vi "PCO_RecorderSaveImage_B16.vi"(0 "pImgBuf":u16[][](array[numeric])=array1x4097[4097 elements], 1 "wWidth":u16, 2 "wHeight":u16, 3 "szFilePath":path, 5 "error in (no error)":errorcluster {"code" format="%x"}, 6 "isColor":bool, 8 "bIsBitmap":bool, 9 "PCO_METADATA_STRUCT":T1={"wVersion"=65535, "dwIMAGE_COUNTER"=0, "dwIMAGE_TIME_US"=0, "lvTimestamp"=timestamp(0 s since 1904-01-01), "bIMAGE_TIME_STATUS"=0, "wEXPOSURE_TIME_BASE"=0, "dwEXPOSURE_TIME"=0, "dwFRAMERATE_MILLIHZ"=0, "sSENSOR_TEMPERATURE"=0, "wIMAGE_SIZE_X"=0, "wIMAGE_SIZE_Y"=0, "bBINNING_X"=0, "bBINNING_Y"=0, "dwSENSOR_READOUT_FREQUENCY"=0, "wSENSOR_CONV_FACTOR"=0, "dwCAMERA_SERIAL_NO"=0, "wCAMERA_TYPE"=0, "bBIT_RESOLUTION"=0, "bSYNC_STATUS"=0, "wDARK_OFFSET"=0, "bTRIGGER_MODE"=0, "bDOUBLE_IMAGE_MODE"=0, "bCAMERA_SYNC_MODE"=0, "bIMAGE_TYPE"=0, "wCOLOR_PATTERN"=0, "wCAMERA_SUBTYPE"=0, "dwEVENT_NUMBER"=0, "wIMAGE_SIZE_X_Offset"=0, "wIMAGE_SIZE_Y_Offset"=0}, 10 "bOverwrite":bool) -> (14 "ErrorMessage":i32 format="%x", 19 "error out":errorcluster {"code" format="%x"})   [LabVIEW 2019, in "Recorder.lvlib"]
doc: "int WINAPI PCO_RecorderSaveImage(void* pImgBuf, WORD wWidth, WORD wHeight, const char* cFileType, bool bIsBitmap, const char* szFilePath, bool bOverwrite, PCO_METADATA_STRUCT* strMetadata);"
uses:
  Recorder.lvlib
  pco.sdk/Structures/Structures.lvlib
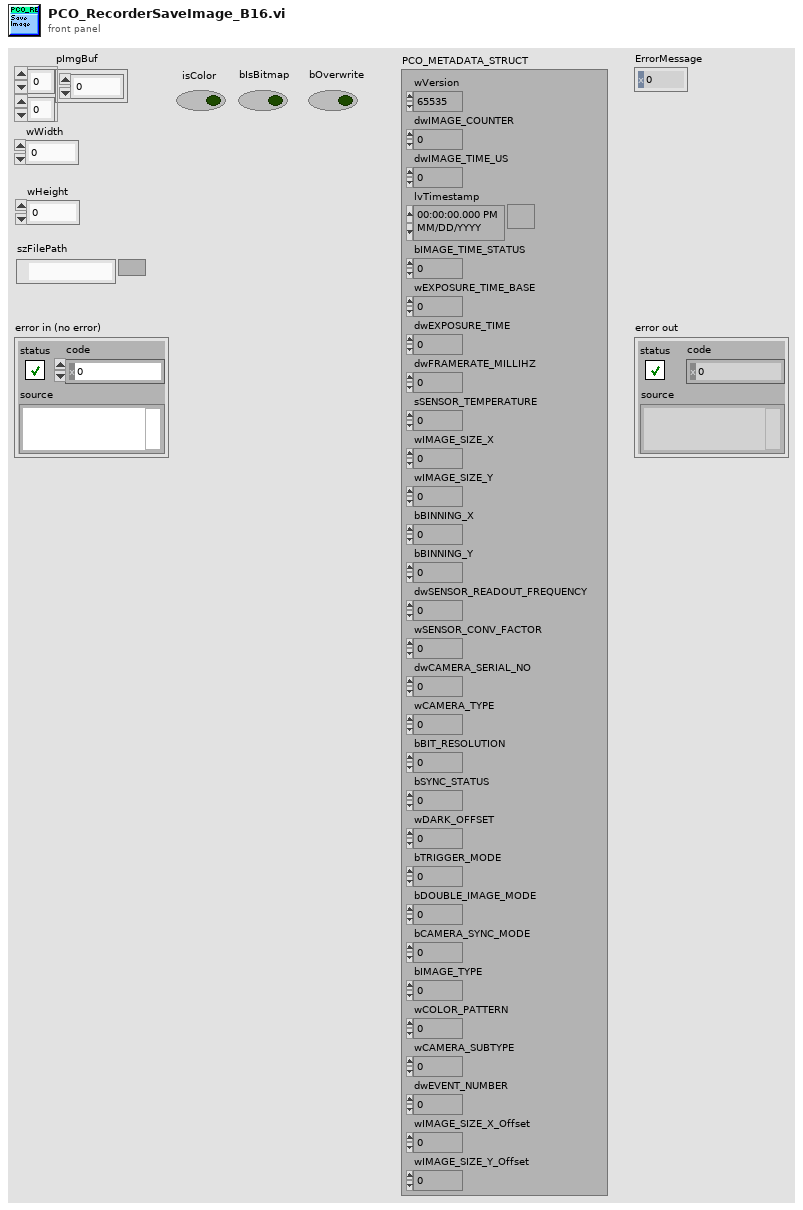
[diagram p1: front panel]
types:
  T1 = cluster{"wVersion":u16, "dwIMAGE_COUNTER":u32, "dwIMAGE_TIME_US":u32, "lvTimestamp":timestamp, "bIMAGE_TIME_STATUS":u8, "wEXPOSURE_TIME_BASE":u16, "dwEXPOSURE_TIME":u32, "dwFRAMERATE_MILLIHZ":u32, "sSENSOR_TEMPERATURE":i16, "wIMAGE_SIZE_X":u16, "wIMAGE_SIZE_Y":u16, "bBINNING_X":u8, "bBINNING_Y":u8, "dwSENSOR_READOUT_FREQUENCY":u32, "wSENSOR_CONV_FACTOR":u16, "dwCAMERA_SERIAL_NO":u32, "wCAMERA_TYPE":u16, "bBIT_RESOLUTION":u8, "bSYNC_STATUS":u8, "wDARK_OFFSET":u16, "bTRIGGER_MODE":u8, "bDOUBLE_IMAGE_MODE":u8, "bCAMERA_SYNC_MODE":u8, "bIMAGE_TYPE":u8, "wCOLOR_PATTERN":u16, "wCAMERA_SUBTYPE":u16, "dwEVENT_NUMBER":u32, "wIMAGE_SIZE_X_Offset":u16, "wIMAGE_SIZE_Y_Offset":u16}
  T2 = typedef "LVDateTimeRec.ctl" = cluster{"fractional second":dbl, "second":i32, "minute":i32, "hour":i32, "day of month":i32, "month":i32, "year":i32, "day of week":i32, "day of year":i32, "DST":i32}
  T3 = cluster{"wSize":u16, "wVersion":u16, "bIMAGE_COUNTER_BCD":cluster{u8, u8, u8, u8}, "bIMAGE_TIME_US_BCD":cluster{u8, u8, u8}, "bIMAGE_TIME_SEC_BCD":u8, "bIMAGE_TIME_MIN_BCD":u8, "bIMAGE_TIME_HOUR_BCD":u8, "bIMAGE_TIME_DAY_BCD":u8, "bIMAGE_TIME_MON_BCD":u8, "bIMAGE_TIME_YEAR_BCD":u8, "bIMAGE_TIME_STATUS":u8, "wEXPOSURE_TIME_BASE":u16, "dwEXPOSURE_TIME":u32, "dwFRAMERATE_MILLIHZ":u32, "sSENSOR_TEMPERATURE":i16, "wIMAGE_SIZE_X":u16, "wIMAGE_SIZE_Y":u16, "bBINNING_X":u8, "bBINNING_Y":u8, "dwSENSOR_READOUT_FREQUENCY":u32, "wSENSOR_CONV_FACTOR":u16, "dwCAMERA_SERIAL_NO":u32, "wCAMERA_TYPE":u16, "bBIT_RESOLUTION":u8, "bSYNC_STATUS":u8, "wDARK_OFFSET":u16, "bTRIGGER_MODE":u8, "bDOUBLE_IMAGE_MODE":u8, "bCAMERA_SYNC_MODE":u8, "bIMAGE_TYPE":u8, "wCOLOR_PATTERN":u16, "wCAMERA_SUBTYPE":u16, "dwEVENT_NUMBER":u32, "wIMAGE_SIZE_X_Offset":u16, "wIMAGE_SIZE_Y_Offset":u16}
  T4 = enum16{"big-endian, network order", "native, host order", "little-endian"}
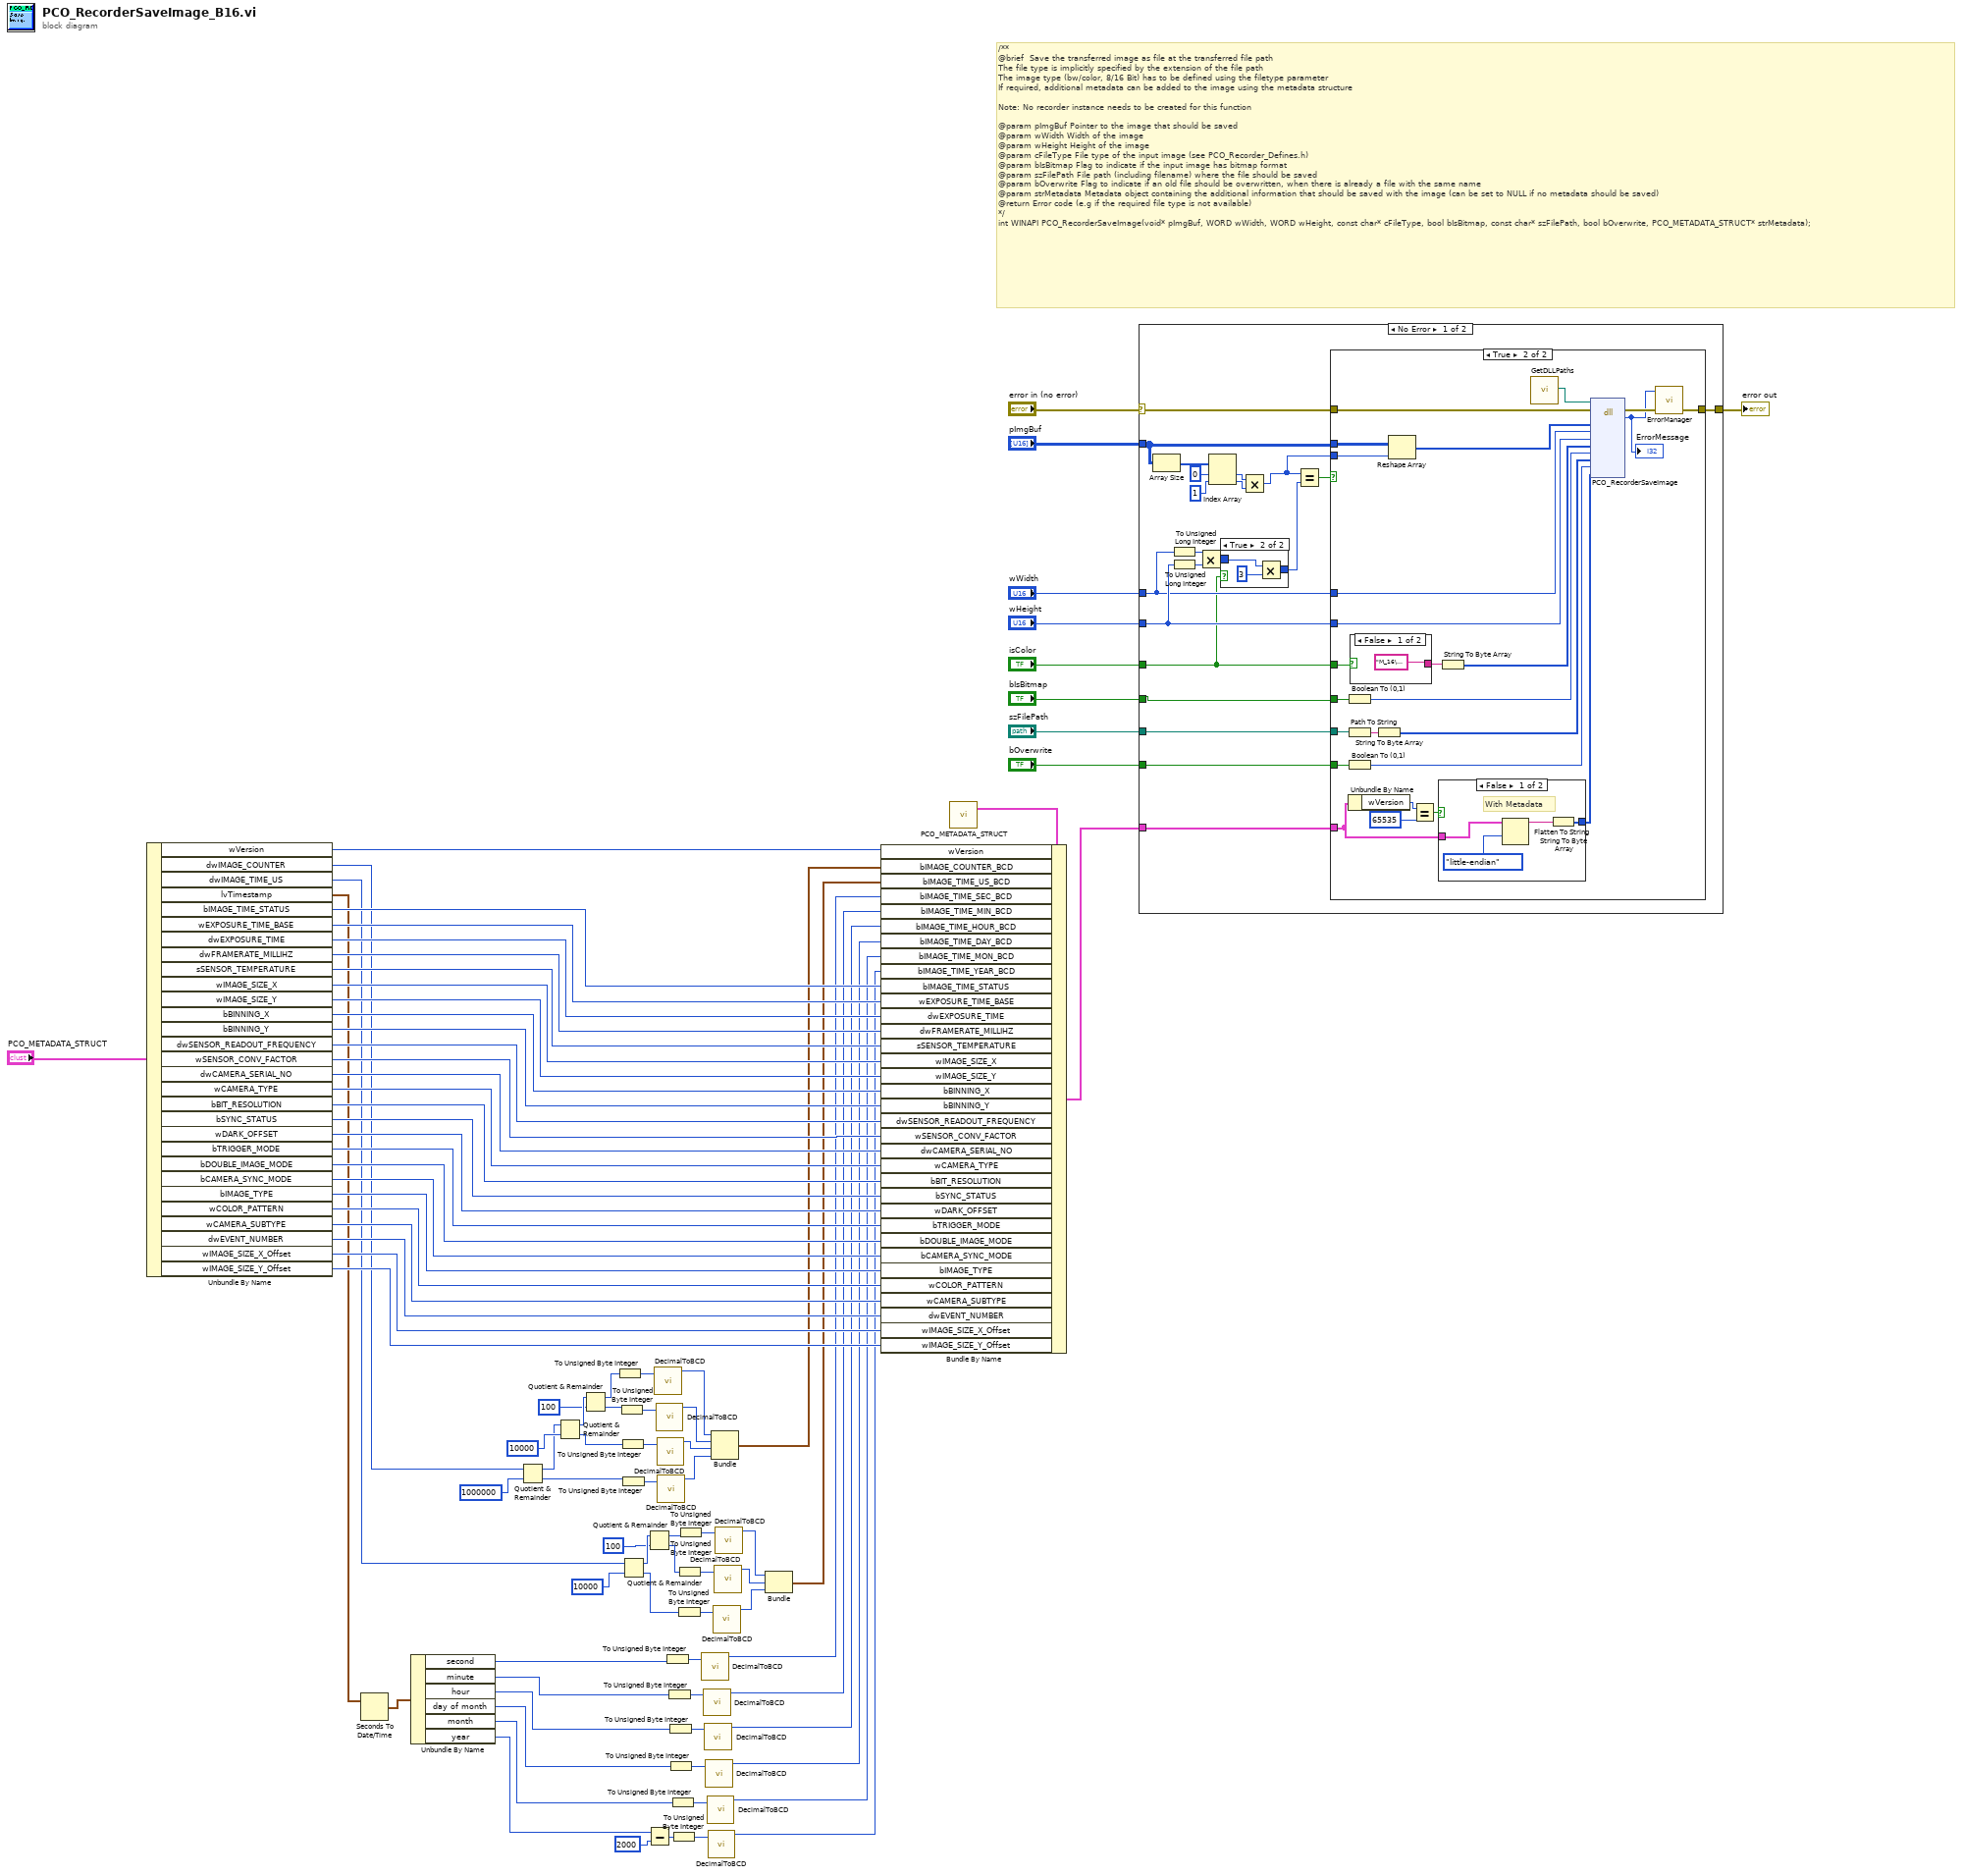
[diagram p0: block diagram]
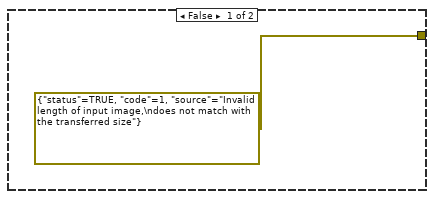
[diagram p3: hidden frame]
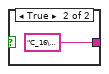
[diagram p4: hidden frame]
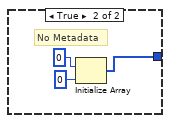
[diagram p5: hidden frame]
diagram:
  # "/**\n@brief  Save the transferred image as file at the transferred file path\nThe file type is implicitly specified by the extension of the file path\nThe image type (bw/color, 8/16 Bit) has to be defined using the filetype parameter\nIf required, additional metadata can be added to the image using the metadata structure\n\nNote: No recorder instance needs to be created for this function\n\n@param pImgBuf Pointer to the image that should be saved\n@param wWidth Width of the image\n@param wHeight Height of the image\n@param cFileType File type of the input image (see PCO_Recorder_Defines.h)\n@param bIsBitmap Flag to indicate if the input image has bitmap format\n@param szFilePath File path (including filename) where the file should be saved\n@param bOverwrite Flag to indicate if an old file should be overwritten, when there is already a file with the same name\n@param strMetadata Metadata object containing the additional information that should be saved with the image (can be set to NULL if no metadata should be saved)\n@return Error code (e.g if the required file type is not available)\n*/\nint WINAPI PCO_RecorderSaveImage(void* pImgBuf, WORD wWidth, WORD wHeight, const char* cFileType, bool bIsBitmap, const char* szFilePath, bool bOverwrite, PCO_METADATA_STRUCT* strMetadata);"
  n1 = Unbundle By Name("PCO_METADATA_STRUCT") -> ("wVersion"=w83:u16, "dwIMAGE_COUNTER"=w17:u32, "dwIMAGE_TIME_US"=w22:u32, "lvTimestamp"=w57:timestamp, "bIMAGE_TIME_STATUS"=w71:u8, "wEXPOSURE_TIME_BASE"=w58:u16, "dwEXPOSURE_TIME"=w59:u32, "dwFRAMERATE_MILLIHZ"=w60:u32, "sSENSOR_TEMPERATURE"=w61:i16, "wIMAGE_SIZE_X"=w62:u16, "wIMAGE_SIZE_Y"=w63:u16, "bBINNING_X"=w64:u8, "bBINNING_Y"=w65:u8, "dwSENSOR_READOUT_FREQUENCY"=w66:u32, "wSENSOR_CONV_FACTOR"=w67:u16, "dwCAMERA_SERIAL_NO"=w68:u32, "wCAMERA_TYPE"=w69:u16, "bBIT_RESOLUTION"=w70:u8, "bSYNC_STATUS"=w72:u8, "wDARK_OFFSET"=w73:u16, "bTRIGGER_MODE"=w74:u8, "bDOUBLE_IMAGE_MODE"=w75:u8, "bCAMERA_SYNC_MODE"=w76:u8, "bIMAGE_TYPE"=w77:u8, "wCOLOR_PATTERN"=w78:u16, "wCAMERA_SUBTYPE"=w79:u16, "dwEVENT_NUMBER"=w80:u32, "wIMAGE_SIZE_X_Offset"=w81:u16, "wIMAGE_SIZE_Y_Offset"=w82:u16)
  n2 = Seconds To Date/Time(time stamp (now)=w57) -> (date time rec=w56:T2)  [unwired: 1 in]
  n3 = Unbundle By Name(w56) -> ("second"=w55:i32, "minute"=w52:i32, "hour"=w47:i32, "day of month"=w46:i32, "month"=w45:i32, "year"=w42:i32)
  n4 = Quotient & Remainder(x=w17, y=u32 1000000 ("x")) -> (x-y*floor(x/y)=w16:u32, floor(x/y)=w11:u32)
  n5 = Quotient & Remainder(x=w16, y=u32 10000 ("x")) -> (x-y*floor(x/y)=w20:u32, floor(x/y)=w10:u32)
  n6 = Quotient & Remainder(x=w20, y=u32 100 ("x")) -> (x-y*floor(x/y)=w8:u32, floor(x/y)=w9:u32)
  n7 = To Unsigned Byte Integer(number=w8) -> (unsigned 8bit integer=w15:u8)
  n8 = To Unsigned Byte Integer(number=w9) -> (unsigned 8bit integer=w14:u8)
  n9 = To Unsigned Byte Integer(number=w10) -> (unsigned 8bit integer=w13:u8)
  n10 = To Unsigned Byte Integer(number=w11) -> (unsigned 8bit integer=w12:u8)
  n11 = Quotient & Remainder(x=w22, y=u32 10000 ("x")) -> (x-y*floor(x/y)=w34:u32, floor(x/y)=w27:u32)
  n12 = Quotient & Remainder(x=w34, y=u32 100 ("x")) -> (x-y*floor(x/y)=w31:u32, floor(x/y)=w29:u32)
  n13 = Subtract(x=w42, y=2000) -> (x-y=w43:i32)
  n14 = call "DecimalToBCD.vi"("U8"=w15) -> ("BCD"=w7:u8)  [unwired: 10 in]
  n15 = call "DecimalToBCD.vi"("U8"=w14) -> ("BCD"=w6:u8)  [unwired: 10 in]
  n16 = call "DecimalToBCD.vi"("U8"=w13) -> ("BCD"=w5:u8)  [unwired: 10 in]
  n17 = call "DecimalToBCD.vi"("U8"=w12) -> ("BCD"=w4:u8)  [unwired: 10 in]
  n18 = To Unsigned Byte Integer(number=w55) -> (unsigned 8bit integer=w54:u8)
  n19 = To Unsigned Byte Integer(number=w52) -> (unsigned 8bit integer=w53:u8)
  n20 = To Unsigned Byte Integer(number=w47) -> (unsigned 8bit integer=w51:u8)
  n21 = To Unsigned Byte Integer(number=w46) -> (unsigned 8bit integer=w48:u8)
  n22 = To Unsigned Byte Integer(number=w45) -> (unsigned 8bit integer=w49:u8)
  n23 = To Unsigned Byte Integer(number=w43) -> (unsigned 8bit integer=w50:u8)
  n24 = To Unsigned Byte Integer(number=w27) -> (unsigned 8bit integer=w28:u8)
  n25 = To Unsigned Byte Integer(number=w29) -> (unsigned 8bit integer=w30:u8)
  n26 = To Unsigned Byte Integer(number=w31) -> (unsigned 8bit integer=w32:u8)
  n27 = call "DecimalToBCD.vi"("U8"=w54) -> ("BCD"=w36:u8)  [unwired: 10 in]
  n28 = call "DecimalToBCD.vi"("U8"=w53) -> ("BCD"=w37:u8)  [unwired: 10 in]
  n29 = call "DecimalToBCD.vi"("U8"=w51) -> ("BCD"=w38:u8)  [unwired: 10 in]
  n30 = call "DecimalToBCD.vi"("U8"=w48) -> ("BCD"=w39:u8)  [unwired: 10 in]
  n31 = call "DecimalToBCD.vi"("U8"=w49) -> ("BCD"=w40:u8)  [unwired: 10 in]
  n32 = call "DecimalToBCD.vi"("U8"=w50) -> ("BCD"=w41:u8)  [unwired: 10 in]
  n33 = Bundle("BCD"=w7, "BCD"=w6, "BCD"=w5, "BCD"=w4) -> (w3:cluster{"BCD":u8, "BCD":u8, "BCD":u8, "BCD":u8})  [unwired: 1 in]
  n34 = call "DecimalToBCD.vi"("U8"=w28) -> ("BCD"=w24:u8)  [unwired: 10 in]
  n35 = call "DecimalToBCD.vi"("U8"=w30) -> ("BCD"=w25:u8)  [unwired: 10 in]
  n36 = call "DecimalToBCD.vi"("U8"=w32) -> ("BCD"=w26:u8)  [unwired: 10 in]
  n37 = Bundle("BCD"=w26, "BCD"=w25, "BCD"=w24) -> (w23:cluster{"BCD":u8, "BCD":u8, "BCD":u8})  [unwired: 1 in]
  n38 = call "PCO_METADATA_STRUCT.vi"() -> ("PCO_METADATA_STRUCT_Raw"=w84:T3)  [unwired: 4 in, 3 out]
  n39 = Bundle By Name(cluster=w84, "wVersion"=w83, "bIMAGE_COUNTER_BCD"=w3, "bIMAGE_TIME_US_BCD"=w23, "bIMAGE_TIME_SEC_BCD"=w36, "bIMAGE_TIME_MIN_BCD"=w37, "bIMAGE_TIME_HOUR_BCD"=w38, "bIMAGE_TIME_DAY_BCD"=w39, "bIMAGE_TIME_MON_BCD"=w40, "bIMAGE_TIME_YEAR_BCD"=w41, "bIMAGE_TIME_STATUS"=w71, "wEXPOSURE_TIME_BASE"=w58, "dwEXPOSURE_TIME"=w59, "dwFRAMERATE_MILLIHZ"=w60, "sSENSOR_TEMPERATURE"=w61, "wIMAGE_SIZE_X"=w62, "wIMAGE_SIZE_Y"=w63, "bBINNING_X"=w64, "bBINNING_Y"=w65, "dwSENSOR_READOUT_FREQUENCY"=w66, "wSENSOR_CONV_FACTOR"=w67, "dwCAMERA_SERIAL_NO"=w68, "wCAMERA_TYPE"=w69, "bBIT_RESOLUTION"=w70, "bSYNC_STATUS"=w72, "wDARK_OFFSET"=w73, "bTRIGGER_MODE"=w74, "bDOUBLE_IMAGE_MODE"=w75, "bCAMERA_SYNC_MODE"=w76, "bIMAGE_TYPE"=w77, "wCOLOR_PATTERN"=w78, "wCAMERA_SUBTYPE"=w79, "dwEVENT_NUMBER"=w80, "wIMAGE_SIZE_X_Offset"=w81, "wIMAGE_SIZE_Y_Offset"=w82) -> (w1:T3)
  n40 = case shown="No Error" "error in (no error)" {
    selector: "error in (no error)" -> [w113 w154]
    tunnel: "pImgBuf" -> [w112 _]
    tunnel: "wWidth" -> [w95 _]
    tunnel: "wHeight" -> [w96 _]
    tunnel: "bIsBitmap" -> [w106 _]
    tunnel: [w114 w154] -> w89
    tunnel: "szFilePath" -> [w107 _]
    tunnel: "bOverwrite" -> [w108 _]
    tunnel: "isColor" -> [w94 _]
    tunnel: w1 -> [w109 _]
    frame No Error {
      n41 = Array Size(array=w112) -> (size(s)=w105:i32[])
      n42 = To Unsigned Long Integer(number=w95) -> (unsigned 32bit integer=w98:u32)
      n43 = To Unsigned Long Integer(number=w96) -> (unsigned 32bit integer=w97:u32)
      n44 = Multiply(x=w98, y=w97) -> (x*y=w111:u32)
      n45 = Index Array(array=w105, index #1=0 ("index"), index #2=1 ("index")) -> (element #1=w103:i32, element #2=w101:i32)
      n46 = case shown="True" w94 {
        tunnel: w111 -> [w115 w118]
        tunnel: [w115 w116] -> w100
        frame False {
        }
        frame True {
          n47 = Multiply(x=w118, y=u16 3) -> (x*y=w116:u32)
        }
      }
      n48 = Multiply(x=w103, y=w101) -> (x*y=w99:i32)
      n49 = Equal?(x=w99, y=w100) -> (x = y?=w110:bool)
      n50 = case shown="True" w110 {
        tunnel: w112 -> [_ w122]
        tunnel: w95 -> [_ w144]
        tunnel: w96 -> [_ w143]
        tunnel: w106 -> [_ w142]
        tunnel: [errorcluster {"status"=TRUE, "code"=1, "source"="Invalid length of input image,\ndoes not match with the transferred size"} ("error out") w136] -> w114
        tunnel: w113 -> [_ w139]
        tunnel: w94 -> [_ w128]
        tunnel: w109 -> [_ w130]
        tunnel: w108 -> [_ w129]
        tunnel: w107 -> [_ w126]
        tunnel: w99 -> [_ w120]
        frame False {
        }
        frame True {
          n51 = Boolean To (0,1)(Boolean=w142) -> (0, 1=w141:i16)
          n52 = Path To String(path=w126) -> (string=w127:string)
          n53 = Boolean To (0,1)(Boolean=w129) -> (0, 1=w140:i16)
          n54 = Unbundle By Name(w130) -> ("wVersion"=w134:u16)
          n55 = case shown="False" w128 {
            tunnel: ["M_16\u0000" "C_16\u0000"] -> w124
            frame False {
            }
            frame True {
            }
          }
          n56 = String To Byte Array(string=w127) -> (unsigned byte array=w125:u8[])
          n57 = Reshape Array(w122, w120) -> (w121:u16[])
          n58 = Equal?(x=w134, y=u16 65535) -> (x = y?=w132:bool)
          n59 = case shown="False" w132 {
            tunnel: [w148 w151] -> w131
            tunnel: w130 -> [w149 _]
            frame False {
              # "With Metadata"
              n60 = Flatten To String(anything=w149, byte order (0:big-endian, network order)=T4."little-endian" ("Byte-Reihenfolge (0:Big-Endian, Netzwerkreihenfolge)")) -> (data string=w150:string)  [unwired: 2 in, 2 out]
              n61 = String To Byte Array(string=w150) -> (unsigned byte array=w148:u8[])
            }
            frame True {
              # "No Metadata"
              n62 = Initialize Array(u8 0, 0 ("dimension size")) -> (w151:u8[])
            }
          }
          n63 = String To Byte Array(string=w124) -> (unsigned byte array=w123:u8[])
          n64 = call "GetDLLPaths.vi"() -> ("PCO_Recorder_Path"=w138:path)  [unwired: 9 in, 2 out]
          n65 = dll-call lib="?" fn="PCO_RecorderSaveImage"(path in=w138, error in=w139, "pImgBuf"=w121, "wWidth"=w144, "wHeight"=w143, "cFileType"=w123, "bIsBitmap"=w141, "szFilePath"=w125, "bOverwrite"=w140, "strMetadata"=w131) -> (error out=w137:errorcluster, "return type"=w135:i32)  [unwired: 9 in, 1 out]
          "ErrorMessage" <- w135
          n66 = call "ErrorManager.vi"("error in (no error)"=w137, "error code"=w135) -> ("error out"=w136:errorcluster)  [unwired: 3 in]
        }
      }
    }
    frame Error {
    }
  }
  "error out" <- w89
